vi "GetPulsePositions.vi"(8 "error in (no error)":errorcluster, 10 "channel name":string, 11 "pulse positions array in":T1[](array[typedef])) -> (0 "error out":errorcluster, 1 "matching pulse positions":T1, 2 "found":bool, 3 "pulse positions array out":T1[](array[typedef]))   [LabVIEW 2017, in "CmsAcquisition.lvlib"]
uses:
  <vilib>/addons/InsightCM/Devices/Shared/Cms/CmsAcquisition/CmsAcquisition.lvlib
  <vilib>/addons/InsightCM/Utilities/Analysis/Shared/controls/PulsePositions.ctl
  <vilib>/addons/InsightCM/Utilities/Analysis/Shared/AnalysisHelper.lvlib
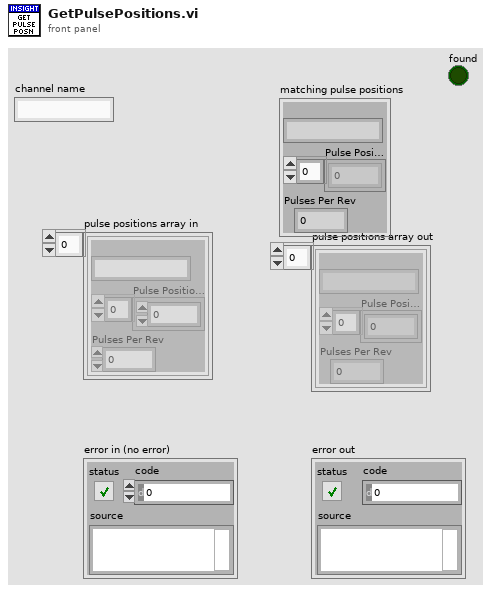
[diagram p1: front panel]
types:
  T1 = typedef "AnalysisHelper.lvlib/PulsePositions.ctl" = cluster{"Name":string, "Pulse Position Data":dbl[], "Pulses Per Rev":i32}
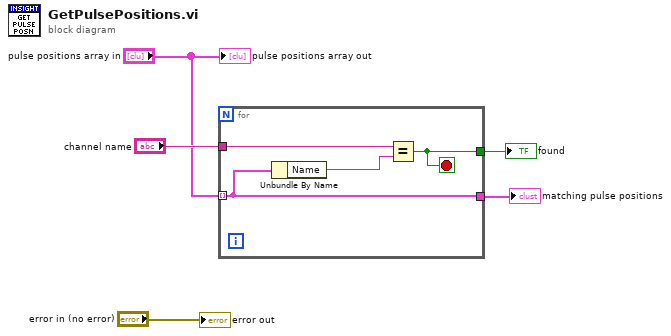
[diagram p0: block diagram]
diagram:
  n1 = for {
    tunnel: "pulse positions array in" -> [w6] mode=indexing
    tunnel: "channel name" -> [w9]
    tunnel: [w8] -> w4
    tunnel: [w6] -> w2
    stop <- w8 stop-if-true
    n2 = Unbundle By Name(w6) -> ("Name"=w7:string)
    n3 = Equal?(x=w9, y=w7) -> (x = y?=w8:bool)
  }
  "found" <- w4
  "matching pulse positions" <- w2
  "pulse positions array out" <- "pulse positions array in"
  "error out" <- "error in (no error)"
